vi "WriteTree.vi"(8 "error in":errorcluster, 11 "repository in":refnum<class "CustomDeviceRepo.lvclass">) -> (0 "error out":errorcluster, 2 "root":T1, 3 "repository out":refnum<class "NISE_CEF_Repository.lvclass">)   [LabVIEW 2019, in "CustomDeviceRepo.lvclass"]
doc: "Transfers information between the repo and the tree control. This method should be called after the custom views are called or saving to disk."
uses:
  CustomDeviceRepo.lvclass
  C:/Program Files (x86)/National Instruments/LabVIEW 2019/vi.lib/NI/Configuration Framework/Repository/NISE_CEF_Repository.lvclass
  <vilib>/NI/Configuration Framework/Repository/NISE_CEF_Repository.lvclass
  <vilib>/NI/Configuration Framework/Node/NodeRef.ctl
  <vilib>/NI/Configuration Framework/Node/NISE_CEF_Node.lvclass
  Custom Device/CustomDevice.lvclass
  <vilib>/NI/Configuration Framework/hierarchy repo/NISE_CEF_HierarchyRepo.lvclass
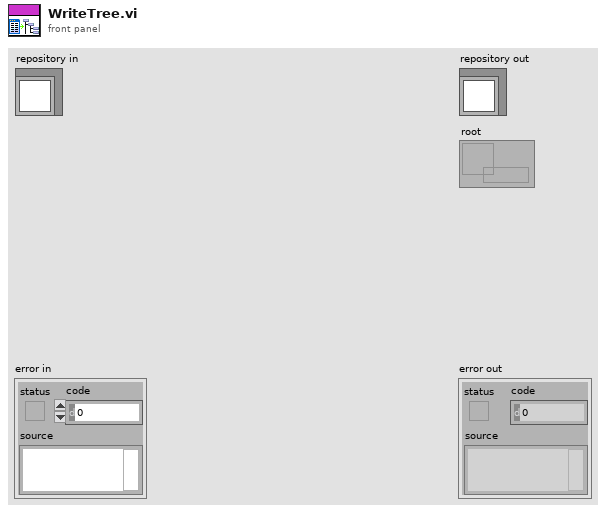
[diagram p1: front panel]
types:
  T1 = typedef "NISE_CEF_Node.lvclass/NodeRef.ctl" = refnum<data-value>
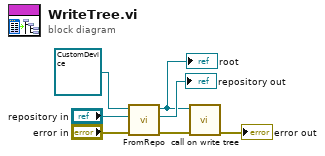
[diagram p0: block diagram]
diagram:
  n1 = call-dynamic "FromRepo.vi"("error in"="error in", "repository in"="repository in", "node in"=refnum<class "CustomDevice.lvclass"> refnum ("CustomDevice.lvclass")) -> ("error out"=w2:errorcluster, "repository out"=→"repository out":refnum<class "NISE_CEF_Repository.lvclass">, "node"=w3:T1)  [unwired: 6 in]
  "root" <- w3
  n2 = call <vilib>:"call on write tree.vi"("error in"=w2, "root"=w3) -> ("error out"=→"error out":errorcluster)  [unwired: 9 in]
